vi "gl_ROI grp window globals.vi"() -> ()   [LabVIEW 2013]
uses:
  Typedefs/ROI grp-window ctrl refs.ctl
panel:
  out "ROI grouping window refresh":bool
  in  "Groups vis window bring to front":bool
  out "Groups vis window refresh":bool
  out "Groups vis window is open":bool
  in  "ZInfo":dbl[](array[numeric])
  out "POI XYZ":dbl[][](array[numeric])
  out "POI Grp Ctrl Refs":T1
  in  "POI Group Indexes []":i32[](array[numeric])
  out "POIArray":i64[][](array[numeric])
  out "ROI grouping window bring to front":bool
  out "ROI grouping window is open":bool
  out "Index of new column":i32
  # "Groups visualisation window"
  # "ROI grouping window"
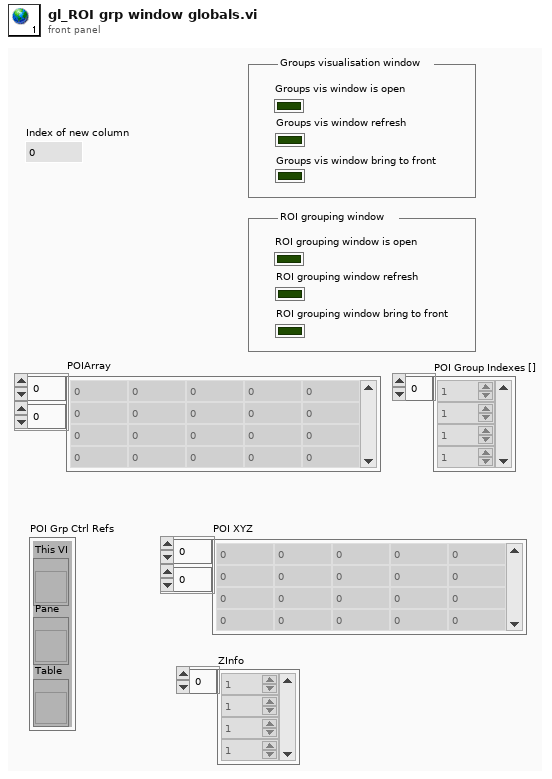
[diagram p1: front panel]
types:
  T1 = typedef "ROI grp-window ctrl refs.ctl" = cluster{"This VI":refnum<vi>, "Pane":refnum<vi>, "Table":refnum<vi>}
diagram:
